vi "MGI Mac Documents Path.vi"(1 "User Documents? (F: Shared Documents)":bool) -> (0 "Path":path)   [LabVIEW 2016]
doc: "Return the path for the User or Shared Documents on the Mac.\n\nAuthored by Shawn D. Walpole\nsupport@mooregoodideas.com\nwww.mooregoodideas.com\n\nCopyright (c) 2010, Moore Good Ideas, Inc.\n\nAll rights reserved.\n\nRedistribution and use in source and binary forms, with or without modification, are permitted provided that the following conditions are met:\n\n * Redistributions of source code must retain the above copyright notice, this list of conditions and the following disclaimer.\n * Redistributions in binary form must reproduce the above copyright notice, this list of conditions and the following disclaimer in the documentation and/or other materials provided with the distribution.\n * Neither the name of Moore Good Ideas, Inc. nor the names of its contributors may be used to endorse or promote products derived from this software without specific prior written permission.\n\nTHIS SOFTWARE IS PROVIDED BY THE COPYRIGHT HOLDERS AND CONTRIBUTORS \"AS IS\" AND ANY EXPRESS OR IMPLIED WARRANTIES, INCLUDING, BUT NOT LIMITED TO, THE IMPLIED WARRANTIES OF MERCHANTABILITY AND FITNESS FOR A PARTICULAR PURPOSE ARE DISCLAIMED. IN NO EVENT SHALL THE COPYRIGHT OWNER OR CONTRIBUTORS BE LIABLE FOR ANY DIRECT, INDIRECT, INCIDENTAL, SPECIAL, EXEMPLARY, OR CONSEQUENTIAL DAMAGES (INCLUDING, BUT NOT LIMITED TO, PROCUREMENT OF SUBSTITUTE GOODS OR SERVICES; LOSS OF USE, DATA, OR PROFITS; OR BUSINESS INTERRUPTION) HOWEVER CAUSED AND ON ANY THEORY OF LIABILITY, WHETHER IN CONTRACT, STRICT LIABILITY, OR TORT (INCLUDING NEGLIGENCE OR OTHERWISE) ARISING IN ANY WAY OUT OF THE USE OF THIS SOFTWARE, EVEN IF ADVISED OF THE POSSIBILITY OF SUCH DAMAGE."
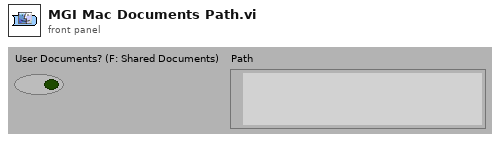
[diagram p1: front panel]
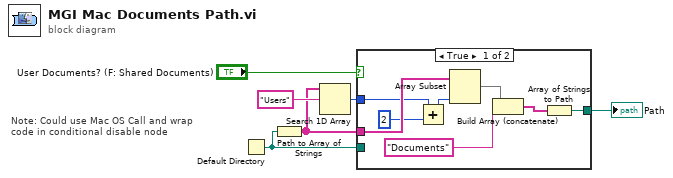
[diagram p0: block diagram]
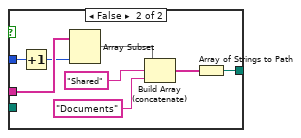
[diagram p2: hidden frame]
diagram:
  # "Note: Could use Mac OS Call and wrap code in conditional disable node"
  n1 = Default Directory() -> (w5:path)
  n2 = Path to Array of Strings(0:w5) -> (2:w3:string[])  [unwired: 1 out]
  n3 = Search 1D Array(1D array=w3, element="Users") -> (index of element=w4:i32)  [unwired: 1 in]
  n4 = case shown="True" "User Documents? (F: Shared Documents)" {
    tunnel: [w14 w22] -> w1
    tunnel: w5 -> [_ _]
    tunnel: w4 -> [w9 w20]
    tunnel: w3 -> [w13 w21]
    frame True {
      n5 = Add(x=w9, y=2) -> (x+y=w8:i32)
      n6 = Array Subset(array=w13, length=w8) -> (w12:string[])  [unwired: 1 in]
      n7 = Build Array (concatenate)(w12, "Documents" ("element")) -> (w10:string[])
      n8 = Array of Strings to Path(0:w10) -> (2:w14:path)  [unwired: 1 in]
    }
    frame False {
      n9 = Increment(x=w20) -> (x+1=w19:i32)
      n10 = Array Subset(array=w21, length=w19) -> (w18:string[])  [unwired: 1 in]
      n11 = Build Array (concatenate)(w18, "Shared" ("element"), "Documents" ("element")) -> (w15:string[])
      n12 = Array of Strings to Path(0:w15) -> (2:w22:path)  [unwired: 1 in]
    }
  }
  "Path" <- w1
